vi "Sub_BuildChannelList.vi"(6 "error in":errorcluster, 7 "iCount":i32, 9 "iStart":i32) -> (0 "error out":errorcluster, 3 "buildChannelList":string)   [LabVIEW 2009]
panel:
  # "Build Channel List"
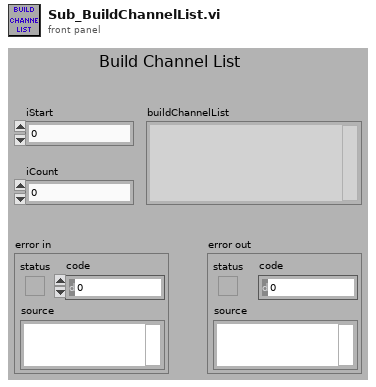
[diagram p1: front panel]
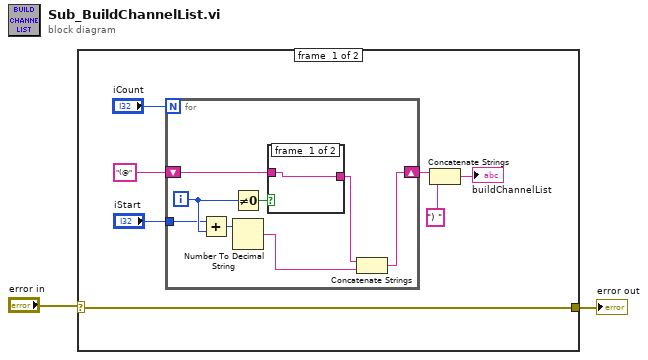
[diagram p0: block diagram]
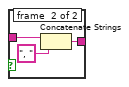
[diagram p2: hidden frame]
diagram:
  n1 = case shown="No Error" "error in" {
    selector: "error in" -> [w3 w22]
    tunnel: [w3 w22] -> w1
    frame #0 {
      n2 = for {
        N: "iCount" -> [_]
        tunnel: "iStart" -> [w16]
        shift-right: [w14] -> w5
        shift-left: "(@" -> [w12]
        i -> [w17]
        n3 = Add(x=w16, y=w17) -> (x+y=w15:i32)
        n4 = Not Equal To 0?(x=w17) -> (x != 0?=w13:bool)
        n5 = Number To Decimal String(number=w15) -> (decimal integer string=w10:string)  [unwired: 1 in]
        n6 = case shown="False" w13 {
          tunnel: w12 -> [w18 w20]
          tunnel: [w18 w19] -> w11
          frame #0 {
          }
          frame #1 {
            n7 = Concatenate Strings(w20, ", " ("string")) -> (w19:string)
          }
        }
        n8 = Concatenate Strings(w11, w10) -> (w14:string)
      }
      n9 = Concatenate Strings(w5, ") " ("string")) -> (→"buildChannelList":string)
    }
    frame #1 {
    }
  }
  "error out" <- w1
